vi "state告警数据存储.vi"(8 "错误输入（无错误）":errorcluster, 10 "data":T1, 11 "state":string) -> (0 "错误输出":errorcluster)   [LabVIEW 2016, in "Alarm interface.lvlib"]
uses:
  Alarm interface.lvlib
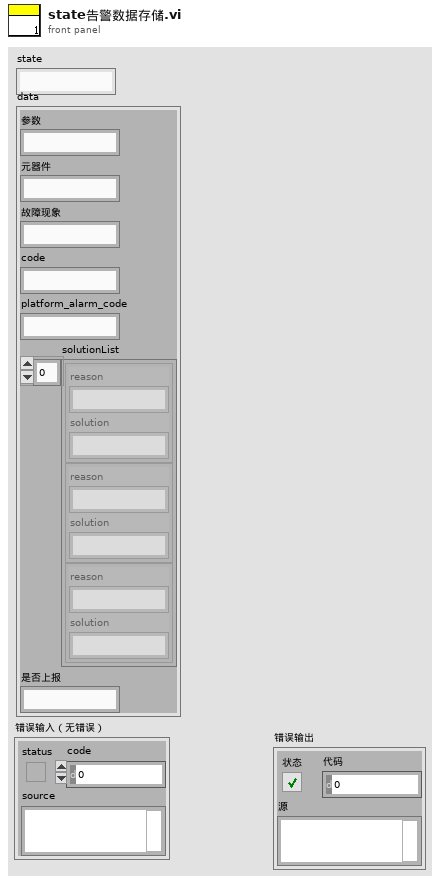
[diagram p1: front panel]
types:
  T1 = typedef "Alarm interface.lvlib/报警短信语音交互.ctl" = cluster{"参数":string, "元器件":string, "故障现象":string, "code":string, "platform_alarm_code":string, "solutionList":cluster{"reason":string, "solution":string}[], "是否上报":string}
  T2 = typedef "报警信息字段定义.ctl" = cluster{"时间":timestamp, "参数":string, "元器件":string, "故障现象":string, "故障分析":string, "state":string, "code":string, "platform_alarm_code":string, "是否上报":string}
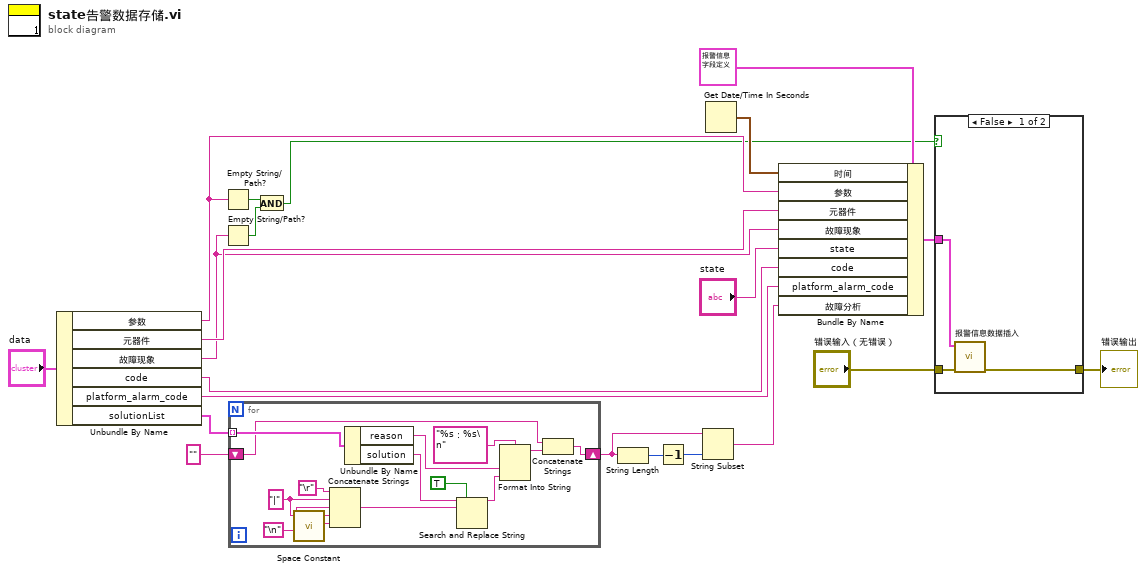
[diagram p0: block diagram]
diagram:
  n1 = Unbundle By Name("data") -> ("参数"=w6:string, "元器件"=w10:string, "故障现象"=w5:string, "code"=w11:string, "platform_alarm_code"=w12:string, "solutionList"=w14:cluster{"reason":string, "solution":string}[])
  n2 = Empty String/Path?(string/path=w6) -> (empty?=w4:bool)
  n3 = Empty String/Path?(string/path=w5) -> (empty?=w3:bool)
  n4 = for {
    tunnel: w14 -> [w35] mode=indexing
    shift-right: [w30] -> w15
    shift-left: "" -> [w31]
    w23 = "|" ("字符串")
    n5 = call <vilib>:"Space Constant.vi"() -> ("String"=w22:string)
    n6 = Concatenate Strings("\r", w23, "\n", w23, w22) -> (w26:string)
    n7 = Unbundle By Name(w35) -> ("reason"=w33:string, "solution"=w29:string)
    n8 = Search and Replace String(replace all?=TRUE ("替换全部？(F)"), input string=w29, search string=w26) -> (result string=w24:string)  [unwired: 5 in, 3 out]
    n9 = Format Into String(format string="%s：%s\n" ("格式字符串"), w33, w24) -> (resulting string=w32:string)  [unwired: 2 in, 1 out]
    n10 = Concatenate Strings(w31, w32) -> (w30:string)
  }
  n11 = And(x=w4, y=w3) -> (x .and. y?=w2:bool)
  n12 = String Length(string=w15) -> (length=w16:i32)
  n13 = Decrement(x=w16) -> (x-1=w17:i32)
  n14 = String Subset(string=w15, length (rest)=w17) -> (substring=w18:string)  [unwired: 1 in]
  n15 = Get Date/Time In Seconds() -> (seconds since 1Jan1904=w9:timestamp)
  n16 = Bundle By Name(cluster=T2 {"时间"=timestamp(0 s since 1904-01-01), "参数"="", "元器件"="", "故障现象"="", "故障分析"="", "state"="", "code"="", "platform_alarm_code"="", "是否上报"=""} ("data"), "时间"=w9, "参数"=w6, "元器件"=w10, "故障现象"=w5, "state"="state", "code"=w11, "platform_alarm_code"=w12, "故障分析"=w18) -> (w1:T2)
  n17 = case shown="False" w2 {
    tunnel: [w36 w39] -> w21
    tunnel: "错误输入（无错误）" -> [w38 w39]
    tunnel: w1 -> [w37 _]
    frame False {
      n18 = call "报警信息数据插入.vi"("data"=w37, "错误输入（无错误）"=w38) -> ("错误输出"=w36:errorcluster)  [unwired: 8 in]
    }
    frame True {
    }
  }
  "错误输出" <- w21
